vi "Contour Convex Hull.vi"(7 "Clockwise? (Default: False)":bool, 8 "error in (no error)":errorcluster, 11 "Points in":T1[](array[typedef])) -> (0 "error out":errorcluster, 3 "Points Out":T1[](array[typedef]))   [LabVIEW 2020, in "g_ar_toolkit.shape.lvlib"]
uses:
  g_ar_toolkit.shape.lvlib
  g_ar_toolkit.common/Image Point (Integer).ctl
  g_ar_toolkit.common/g_ar_toolkit.common.lvlib
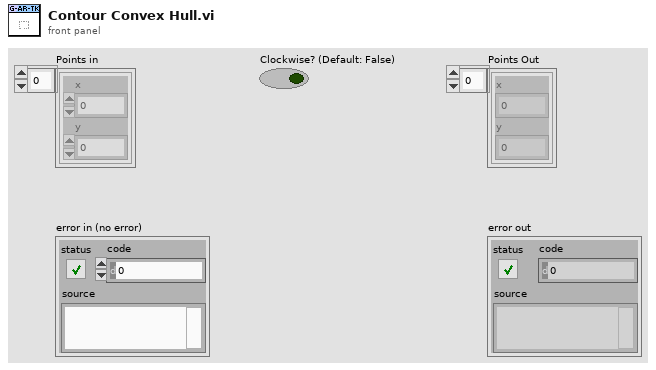
[diagram p1: front panel]
types:
  T1 = typedef "g_ar_toolkit.common.lvlib/Image Point (Integer).ctl" = cluster{"x":i32, "y":i32}
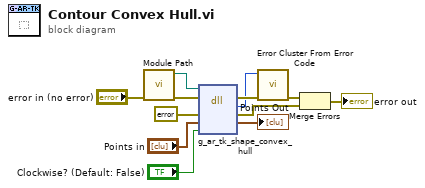
[diagram p0: block diagram]
diagram:
  n1 = call "Module Path.vi"("error in (no error)"="error in (no error)") -> ("error out"=w2:errorcluster, "Path"=w1:path)  [unwired: 9 in]
  n2 = dll-call lib="?" fn="g_ar_tk_shape_convex_hull" ("g_ar_toolkit.*.*:g_ar_tk_image_draw_line")(path in=w1, error in=w2, "error_cluster"=errorcluster {"status"=FALSE, "code"=0, "source"=""} ("error constant"), "points"="Points in", "clockwise"="Clockwise? (Default: False)") -> (error out=w10:errorcluster, "MgErr"=w9:i32, "error_cluster"=w6:errorcluster, "points"=→"Points Out":T1[])  [unwired: 2 in, 1 out]
  n3 = call <vilib>:"Error Cluster From Error Code.vi"("error in (no error)"=w10, "error code (0)"=w9) -> ("error out"=w8:errorcluster)  [unwired: 7 in]
  n4 = Merge Errors(w8, w6) -> (→"error out":errorcluster)
